vi "HO6_Generator3.vi"() -> ()   [LabVIEW 2020]
panel:
  in  "stop":bool
  out "Strip Chart":T1(graph)
  in  "Max":dbl=500.0
  in  "Min":dbl=100.0
  out "When slope is >0, than it's green.":bool
  out "Current Overall average":dbl
  out "Biggest/Smallest value":T2 {"Big time" format="%<%.3X>T"}
  in  "Averaged Points":i16=5 min=1 max=1024 step=1
  in  "?":bool
  in  "Mode":bool
  out "?":enum32{"Iterations", "Timed"}(tab)
  out "Iter Remaining":i32=15
  in  "Iterations to run":i32=10 min=1 step=1
  in  "Time to run (s)":dbl=15.0
  in  "Delay (ms)":i16=500
  out "Countdown (s)":dbl caption="Elapsed Time (s)"
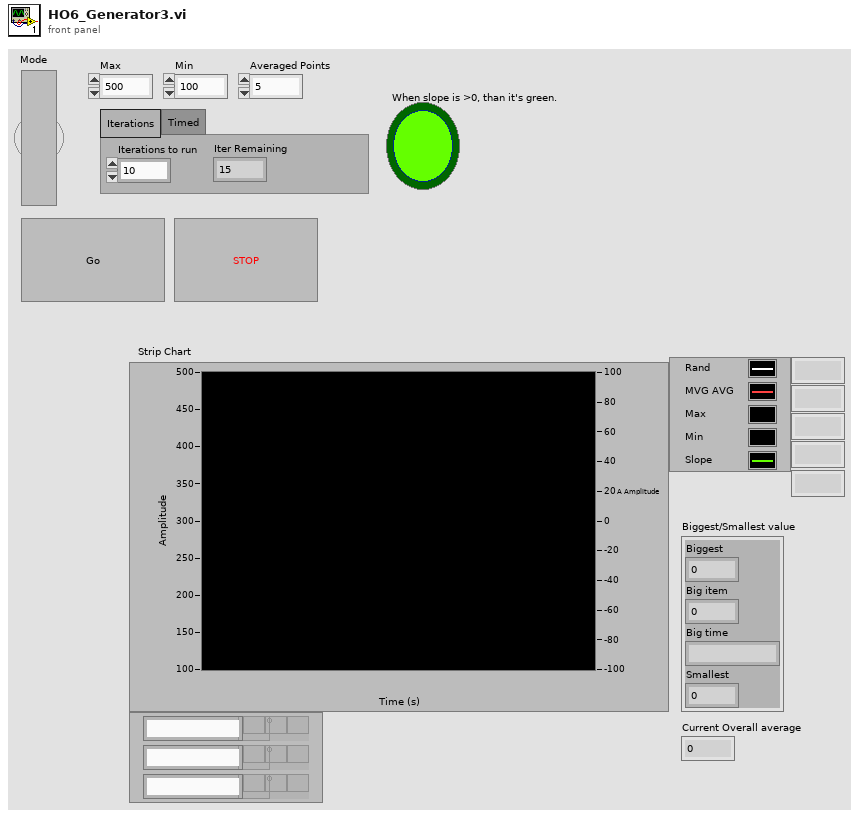
[diagram p1: front panel]
types:
  T1 = cluster{"Double":dbl, dbl, "Max":dbl, "Min":dbl, "Linear Slope":dbl}
  T2 = cluster{"Biggest":dbl, "Big item":i32, "Big time":timestamp, "Smallest":dbl}
  T3 = cluster{"Double":dbl, dbl, "Max":dbl, "Min":dbl, "Linear Slope":dbl}[]
  T4 = cluster{"Double":dbl, dbl, "Max":dbl, "Min":dbl, "Theta (degree)":dbl}
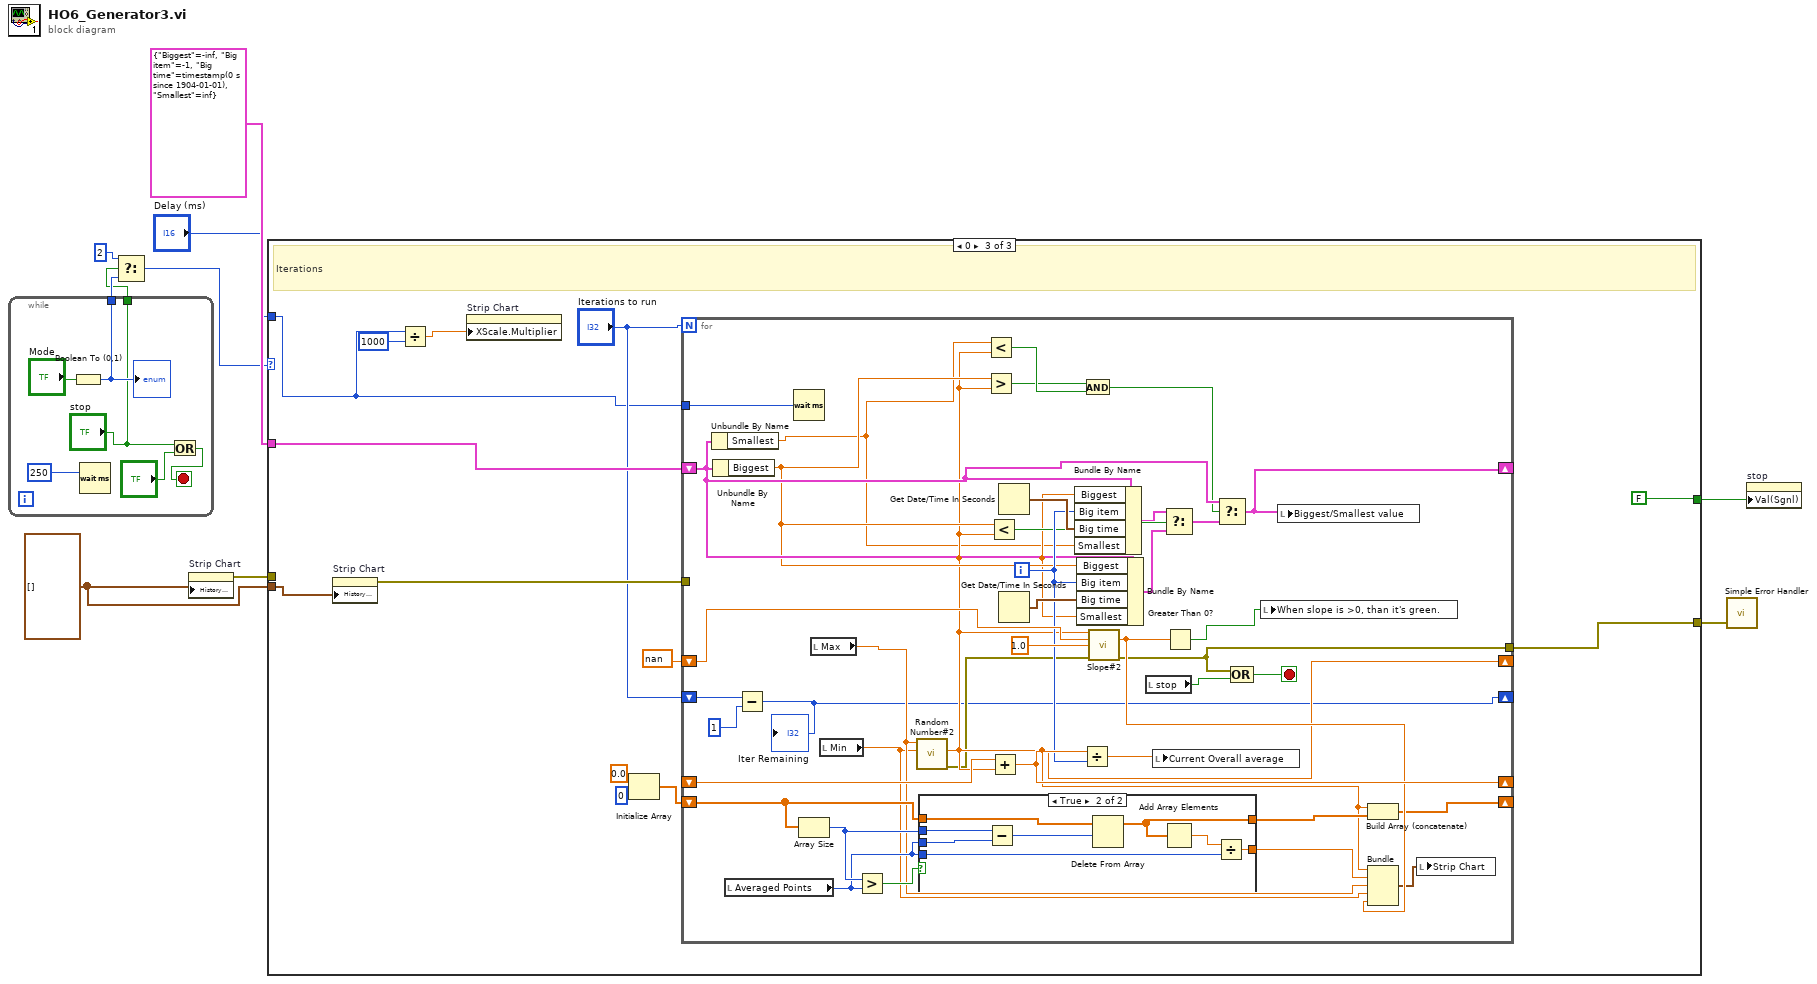
[diagram p0: block diagram]
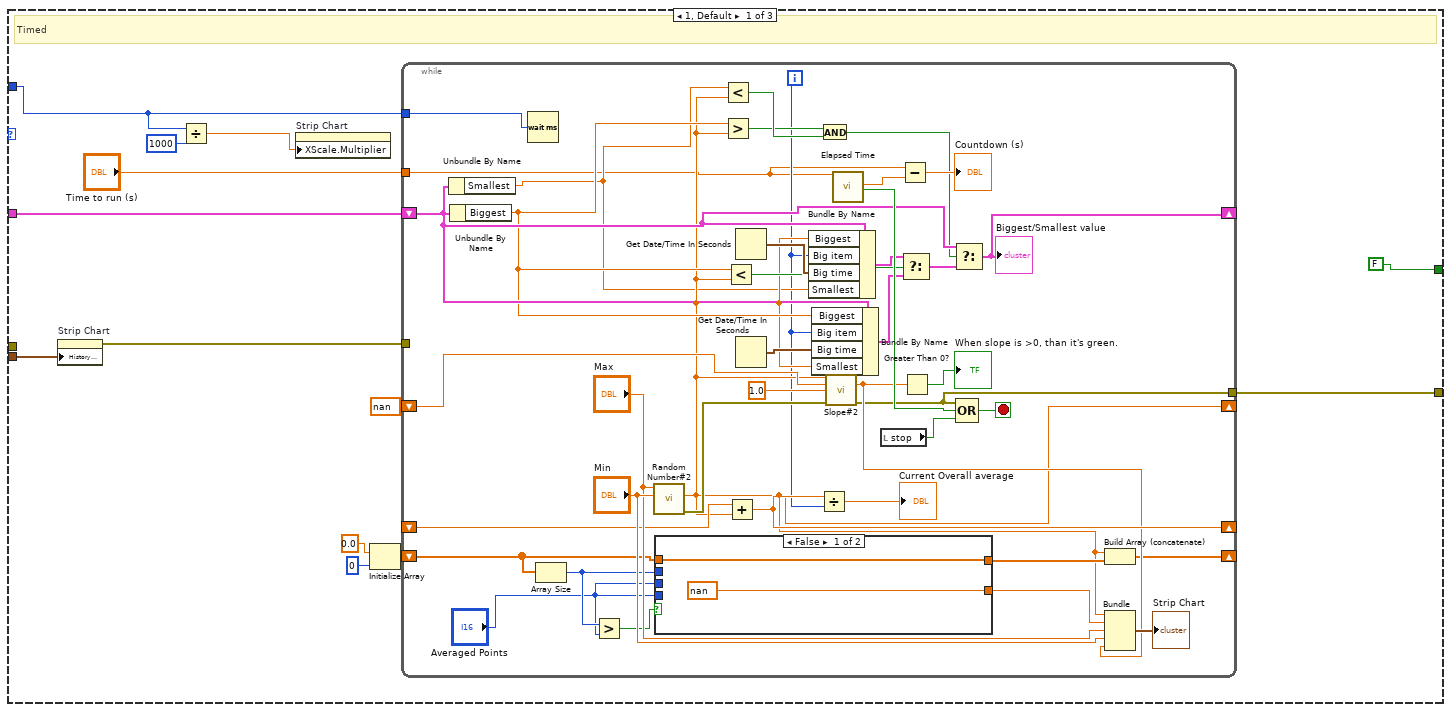
[diagram p2: hidden frame]
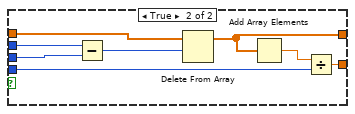
[diagram p3: hidden frame]
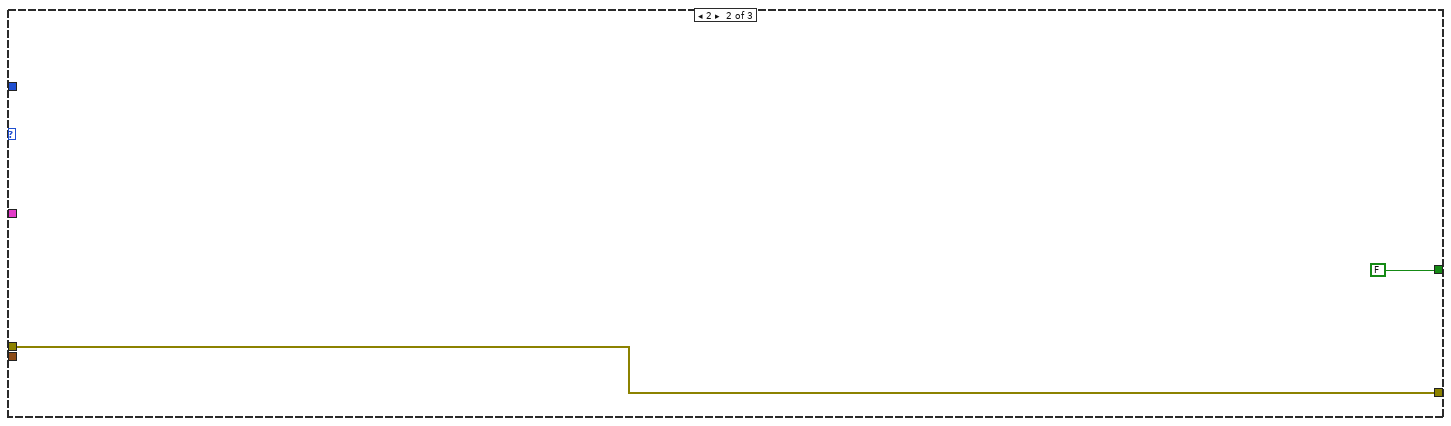
[diagram p4: hidden frame]
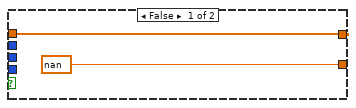
[diagram p5: hidden frame]
diagram:
  w9 = T3 [] ("History Data")
  n1 = while {
    tunnel: [w12] -> w6
    tunnel: ["stop"] -> w2
    stop <- w14 stop-if-true
    n2 = Boolean To (0,1)(Boolean="Mode") -> (0, 1=w12:i16)
    "?" <- w12
    n3 = Wait (ms)(milliseconds to wait=u32 250 ("millisecond timer value")) -> ()  [unwired: 1 out]
    n4 = Or(x="stop", y="?") -> (x .or. y?=w14:bool)
  }
  n5 = Select(t=i16 2, s=w2, f=w6) -> (s? t:f=w5:i16)
  n6 = property on="Strip Chart" class="WFChart (strict)"("History Data"=w9) -> (error out=w3:errorcluster)  [unwired: 2 in, 1 out]
  n7 = case shown="0" w5 {
    tunnel: T2 {"Biggest"=-inf, "Big item"=-1, "Big time"=timestamp(0 s since 1904-01-01), "Smallest"=inf} -> [w24 _ w91]
    tunnel: w9 -> [w23 _ w89]
    tunnel: [w22 w82 w90] -> w8
    tunnel: "Delay (ms)" -> [w21 _ w86]
    tunnel: w3 -> [_ w82 _]
    tunnel: [FALSE FALSE FALSE] -> w1
    frame 1, Default {
      # "Timed"
      n8 = property on="Strip Chart" class="WFChart (strict)"("History Data"=w23) -> (error out=w28:errorcluster)  [unwired: 2 in, 1 out]
      n9 = Divide(x=w21, y=i16 1000) -> (x/y=w18:dbl)
      n10 = property on="Strip Chart" class="WFChart (strict)"("XScale.Multiplier"=w18) -> ()  [unwired: 2 in, 2 out]
      n11 = Initialize Array(0.0 ("element"), 0 ("dimension size")) -> (w29:dbl[])
      n12 = while {
        tunnel: w28 -> [_]
        shift-right: [w64] -> _
        shift-left: _ -> [w65]
        tunnel: [w57] -> w22
        shift-right: [w38] -> _
        shift-left: nan -> [w56]
        shift-right: [w54] -> _
        shift-left: w24 -> [w51]
        shift-right: [w45] -> _
        shift-left: w29 -> [w43]
        tunnel: "Time to run (s)" -> [w31]
        tunnel: w21 -> [w32]
        i -> [w33]
        stop <- w63 stop-if-true
        n13 = Unbundle By Name(w51) -> ("Smallest"=w37:dbl)
        n14 = Unbundle By Name(w51) -> ("Biggest"=w39:dbl)
        n15 = Wait (ms)(milliseconds to wait=w32) -> ()  [unwired: 1 out]
        n16 = Array Size(array=w43) -> (size(s)=w42:i32)
        n17 = Greater?(x=w42, y="Averaged Points") -> (0:w44:bool)
        n18 = call "Random Number#2.vi"("Maximum"="Max", "Minimum"="Min") -> ("Double"=w38:dbl, "error out"=w58:errorcluster)  [unwired: 4 in, 2 out]
        n19 = case shown="False" w44 {
          tunnel: w43 -> [w72 w80]
          tunnel: w42 -> [_ w78]
          tunnel: "Averaged Points" -> [_ w77]
          tunnel: "Averaged Points" -> [_ w76]
          tunnel: [nan w75] -> w41
          tunnel: [w72 w73] -> w40
          frame False {
          }
          frame True {
            n20 = Subtract(x=w78, y=w77) -> (x-y=w79:i32)
            n21 = Delete From Array(array=w80, length=w79) -> (array with subset deleted=w73:dbl[])  [unwired: 1 in, 1 out]
            n22 = Add Array Elements(numeric array=w73) -> (sum=w74:dbl)
            n23 = Divide(x=w74, y=w76) -> (x/y=w75:dbl)
          }
        }
        n24 = Less?(x=w37, y=w38) -> (x < y?=w50:bool)
        n25 = Greater?(x=w39, y=w38) -> (0:w47:bool)
        n26 = Less?(x=w39, y=w38) -> (x < y?=w46:bool)
        n27 = Add(x=w65, y=w38) -> (x+y=w64:dbl)
        n28 = Get Date/Time In Seconds() -> (seconds since 1Jan1904=w53:timestamp)
        n29 = Get Date/Time In Seconds() -> (seconds since 1Jan1904=w52:timestamp)
        n30 = Bundle By Name(cluster=w51, "Biggest"=w38, "Big item"=w33, "Big time"=w53, "Smallest"=w37) -> (w35:T2)
        n31 = Bundle By Name(cluster=w51, "Biggest"=w39, "Big item"=w33, "Big time"=w52, "Smallest"=w38) -> (w36:T2)
        n32 = Divide(x=w64, y=w33) -> (x/y=→"Current Overall average":dbl)
        n33 = And(x=w47, y=w50) -> (x .and. y?=w49:bool)
        n34 = call "Slope#2.vi"("Y2"=w38, "Y1"=w56, "X2 (1)"=1.0, "error in (no error)"=w58) -> ("Theta (degree)"=w59:dbl, "error out"=w57:errorcluster)  [unwired: 8 in, 2 out]
        n35 = call "Elapsed Time"("Time Target (s)"=w31) -> ("Elapsed Time (s)"=w61:dbl, "Time has Elapsed"=w62:bool)  [unwired: 11 in, 6 out]
        n36 = local read "stop"() -> (w30:bool)
        n37 = Subtract(x=w31, y=w61) -> (x-y=→"Countdown (s)":dbl)
        n38 = Select(t=w35, s=w46, f=w36) -> (s? t:f=w48:T2)
        n39 = Greater Than 0?(x=w59) -> (x > 0?=→"When slope is >0, than it's green.":bool)
        n40 = Select(t=w51, s=w49, f=w48) -> (s? t:f=w54:T2)
        "Biggest/Smallest value" <- w54
        n41 = Compound Arithmetic op=OR(w57, w62, w30) -> (w63:bool)
        n42 = Build Array (concatenate)(w38, w40) -> (w45:dbl[])
        n43 = Bundle("Double"=w38, w41, "Max"="Max", "Min"="Min", "Theta (degree)"=w59) -> (→"Strip Chart":T4)  [unwired: 1 in]
      }
    }
    frame 2 {
    }
    frame 0 {
      # "Iterations"
      n44 = property on="Strip Chart" class="WFChart (strict)"("History Data"=w89) -> (error out=w88:errorcluster)  [unwired: 2 in, 1 out]
      n45 = Divide(x=w86, y=i16 1000) -> (x/y=w84:dbl)
      n46 = property on="Strip Chart" class="WFChart (strict)"("XScale.Multiplier"=w84) -> ()  [unwired: 2 in, 2 out]
      n47 = Initialize Array(0.0 ("element"), 0 ("dimension size")) -> (w95:dbl[])
      n48 = for {
        N: "Iterations to run" -> [_]
        shift-right: [w134] -> _
        shift-left: _ -> [w135]
        tunnel: [w98] -> w90
        shift-right: [w114] -> _
        shift-left: nan -> [w132]
        shift-right: [w110] -> _
        shift-left: w91 -> [w127]
        shift-right: [w121] -> _
        shift-left: w95 -> [w119]
        tunnel: w88 -> [_]
        shift-right: [w100] -> _
        shift-left: "Iterations to run" -> [w102]
        tunnel: w86 -> [w99]
        i -> [w128]
        stop <- w96 stop-if-true
        n49 = Unbundle By Name(w127) -> ("Smallest"=w113:dbl)
        n50 = Unbundle By Name(w127) -> ("Biggest"=w115:dbl)
        n51 = local read "Averaged Points"() -> (w107:i16)
        n52 = Subtract(x=w102, y=1) -> (x-y=w100:i32)
        "Iter Remaining" <- w100
        n53 = Wait (ms)(milliseconds to wait=w99) -> ()  [unwired: 1 out]
        n54 = Array Size(array=w119) -> (size(s)=w118:i32)
        n55 = local read "Max"() -> (w106:dbl)
        n56 = local read "Min"() -> (w105:dbl)
        n57 = Greater?(x=w118, y=w107) -> (0:w120:bool)
        n58 = call "Random Number#2.vi"("Maximum"=w106, "Minimum"=w105) -> ("Double"=w114:dbl, "error out"=w103:errorcluster)  [unwired: 4 in, 2 out]
        n59 = case shown="True" w120 {
          tunnel: w119 -> [w137 w145]
          tunnel: w118 -> [_ w143]
          tunnel: w107 -> [_ w142]
          tunnel: w107 -> [_ w141]
          tunnel: [nan w140] -> w117
          tunnel: [w137 w138] -> w116
          frame False {
          }
          frame True {
            n60 = Subtract(x=w143, y=w142) -> (x-y=w144:i32)
            n61 = Delete From Array(array=w145, length=w144) -> (array with subset deleted=w138:dbl[])  [unwired: 1 in, 1 out]
            n62 = Add Array Elements(numeric array=w138) -> (sum=w139:dbl)
            n63 = Divide(x=w139, y=w141) -> (x/y=w140:dbl)
          }
        }
        n64 = Less?(x=w113, y=w114) -> (x < y?=w126:bool)
        n65 = Greater?(x=w115, y=w114) -> (0:w123:bool)
        n66 = Less?(x=w115, y=w114) -> (x < y?=w122:bool)
        n67 = Add(x=w135, y=w114) -> (x+y=w134:dbl)
        n68 = Get Date/Time In Seconds() -> (seconds since 1Jan1904=w130:timestamp)
        n69 = Get Date/Time In Seconds() -> (seconds since 1Jan1904=w129:timestamp)
        n70 = Bundle By Name(cluster=w127, "Biggest"=w114, "Big item"=w128, "Big time"=w130, "Smallest"=w113) -> (w111:T2)
        n71 = Bundle By Name(cluster=w127, "Biggest"=w115, "Big item"=w128, "Big time"=w129, "Smallest"=w114) -> (w112:T2)
        n72 = Divide(x=w134, y=w128) -> (x/y=w109:dbl)
        n73 = And(x=w123, y=w126) -> (x .and. y?=w125:bool)
        n74 = call "Slope#2.vi"("Y2"=w114, "Y1"=w132, "X2 (1)"=1.0, "error in (no error)"=w103) -> ("Theta (degree)"=w133:dbl, "error out"=w98:errorcluster)  [unwired: 8 in, 2 out]
        n75 = local read "stop"() -> (w97:bool)
        n76 = local write "Current Overall average"(w109) -> ()
        n77 = Select(t=w111, s=w122, f=w112) -> (s? t:f=w124:T2)
        n78 = Greater Than 0?(x=w133) -> (x > 0?=w108:bool)
        n79 = Select(t=w127, s=w125, f=w124) -> (s? t:f=w110:T2)
        n80 = Compound Arithmetic op=OR(w98, w97) -> (w96:bool)
        n81 = local write "When slope is >0, than it's green."(w108) -> ()
        n82 = local write "Biggest/Smallest value"(w110) -> ()
        n83 = Build Array (concatenate)(w114, w116) -> (w121:dbl[])
        n84 = Bundle("Double"=w114, w117, "Max"=w106, "Min"=w105, "Theta (degree)"=w133) -> (w104:T4)  [unwired: 1 in]
        n85 = local write "Strip Chart"(w104) -> ()
      }
    }
  }
  n86 = call <vilib>:"Simple Error Handler.vi"("error in (no error)"=w8) -> ()  [unwired: 4 in, 5 out]
  n87 = property on="stop" class="Bool (strict)"("Val(Sgnl)"=w1) -> ()  [unwired: 2 in, 2 out]
